vi "Hub Write.vi"(8 "error in (no error)":errorcluster, 9 "hub port":u64=2, 10 "data in":string, 11 "RP Instrument in":refnum<class "RP Instrument.lvclass">) -> (0 "error out":errorcluster, 3 "RP Instrument out":refnum<class "RP Instrument.lvclass">)   [LabVIEW 2024, in "RP Instrument.lvclass"]
uses:
  RP Instrument.lvclass
  RP Instrument.lvclass/RP Instrument.ctl
  RP Communicator/RP Communicator.lvclass
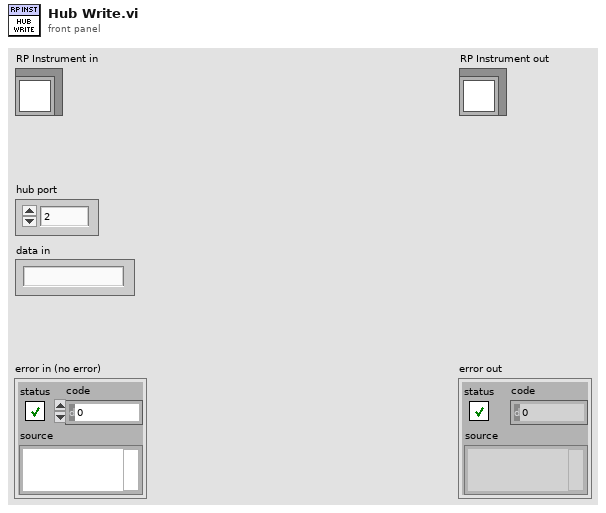
[diagram p1: front panel]
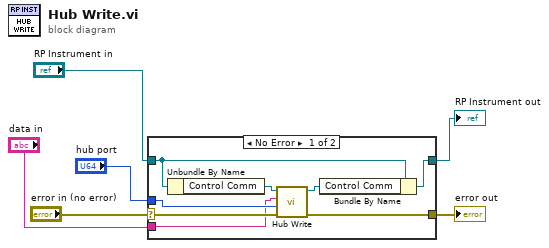
[diagram p0: block diagram]
diagram:
  n1 = case shown="No Error" "error in (no error)" {
    selector: "error in (no error)" -> [w12 w16]
    tunnel: [w11 w16] -> w5
    tunnel: [w10 w15] -> w3
    tunnel: "RP Instrument in" -> [w14 w15]
    tunnel: "hub port" -> [w8 _]
    tunnel: "data in" -> [w7 _]
    frame No Error {
      n2 = Unbundle By Name(w14) -> ("Control Comm"=w13:refnum<class "RP Communicator.lvclass">)
      n3 = call-dynamic "Hub Write.vi"("error in (no error)"=w12, "hub port"=w8, "data in"=w7, "RP Communicator in"=w13) -> ("error out"=w11:errorcluster, "RP Communicator out"=w9:refnum<class "RP Communicator.lvclass">)  [unwired: 6 in]
      n4 = Bundle By Name(cluster=w14, "Control Comm"=w9) -> (w10:refnum<class "RP Instrument.lvclass">)
    }
    frame Error {
    }
  }
  "error out" <- w5
  "RP Instrument out" <- w3
